vi "Brownout Delay Timing.vi"(7 "Waveform Array":waveform(dbl)[](array[waveform])) -> (8 "EdgeDelay":dbl)   [LabVIEW 2010]
uses:
  <vilib>/measure/mamon.llb/Trigger Detection for 1 Channel.vi
  <vilib>/measure/NI_MAPro.lvlib
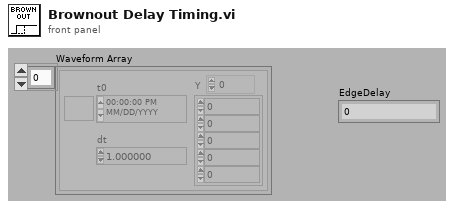
[diagram p1: front panel]
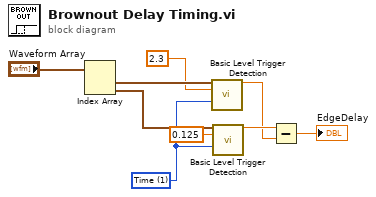
[diagram p0: block diagram]
diagram:
  w5 = u16 1 items=["Index", "Time"] ("location mode")
  n1 = Index Array(array="Waveform Array") -> (element #1=w8:waveform(dbl), element #2=w7:waveform(dbl))  [unwired: 2 in]
  n2 = call-poly <vilib>:"Basic Level Trigger Detection.vi"("signal in"=w8, "level"=2.3, "location mode"=w5) -> ("trigger location"=w3:dbl)  [unwired: 10 in, 2 out]
  n3 = call-poly <vilib>:"Basic Level Trigger Detection.vi"("signal in"=w7, "level"=0.125, "location mode"=w5) -> ("trigger location"=w4:dbl)  [unwired: 10 in, 2 out]
  n4 = Subtract(x=w4, y=w3) -> (x-y=→"EdgeDelay":dbl)
